vi "Stop on Error.vi"(8 "error in":errorcluster, 11 "reference":refnum<vi>) -> (0 "error out":errorcluster, 2 "error?":bool)   [LabVIEW 2012]
uses:
  <vilib>/Utility/error.llb/DialogType.ctl
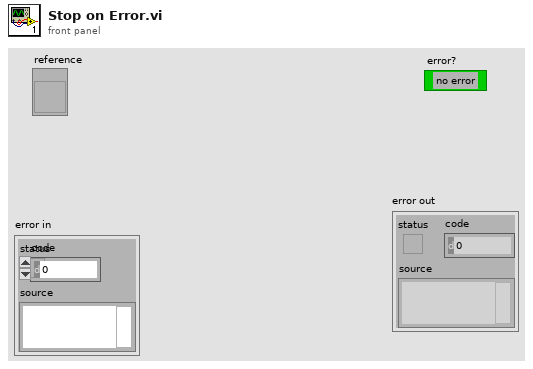
[diagram p1: front panel]
types:
  T1 = typedef "DialogType.ctl" = u16
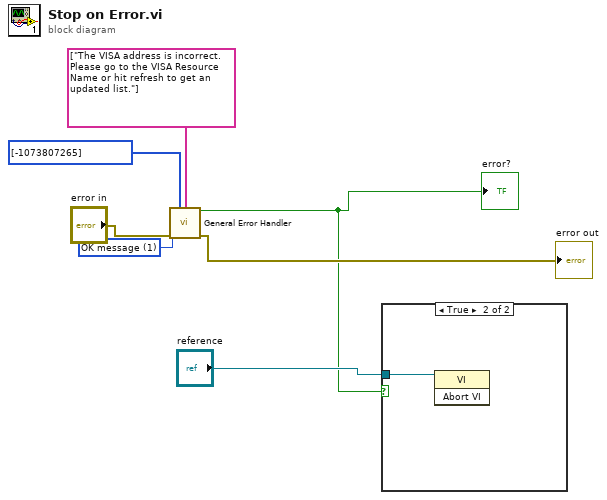
[diagram p0: block diagram]
diagram:
  w6 = T1 1 items=["no dialog", "OK message", "continue or stop message", "OK message + warnings", "continue/stop + warnings"] ("type of dialog (OK msg:1)")
  n1 = call <vilib>:"General Error Handler.vi"("[user-defined codes]"=i32[] [-1073807265], "[user-defined descriptions]"=string[] ["The VISA address is incorrect. Please go to the VISA Resource Name or hit refresh to get an updated list."], "type of dialog (OK msg:1)"=w6, "error in (no error)"="error in") -> ("error?"=w1:bool, "error out"=→"error out":errorcluster)  [unwired: 7 in, 3 out]
  "error?" <- w1
  n2 = case shown="True" w1 {
    tunnel: "reference" -> [_ w8]
    frame False {
    }
    frame True {
      n3 = invoke class="VI" method="Abort VI"(reference=w8) -> ()  [unwired: 2 in, 3 out]
    }
  }
